vi "subpixel_maximum.vi"(1 "Padding":i32=3, 2 "Marginal":dbl[](graph)) -> (0 "Maximum":dbl format="%.2f")   [LabVIEW 2010]
panel:
  out "subpixel part":dbl(graph)
  out "max":dbl(graph)
  out "extracted region":dbl[](graph)
  out "alpha":dbl
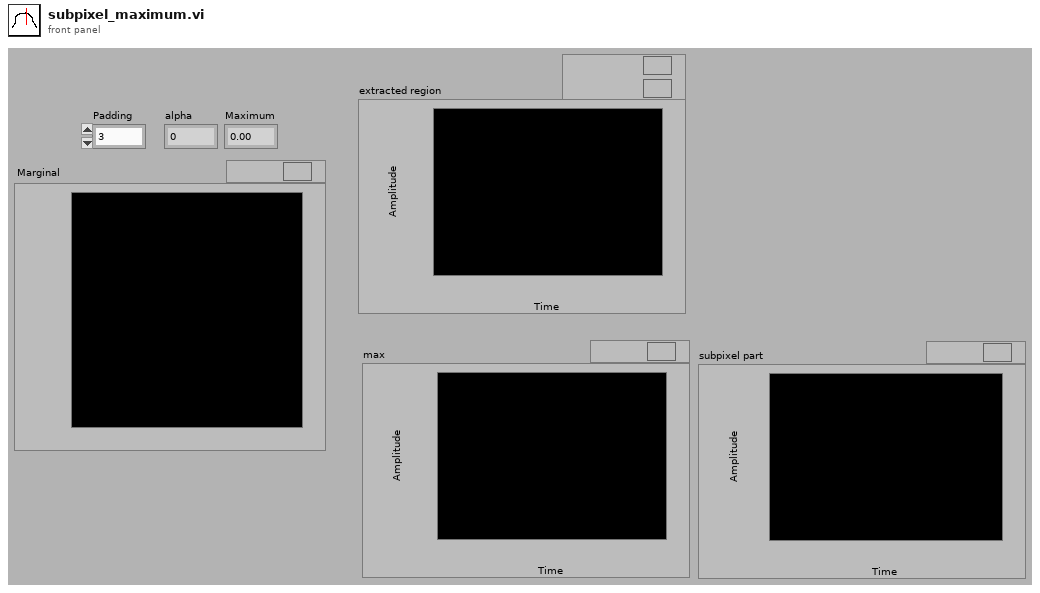
[diagram p1: front panel]
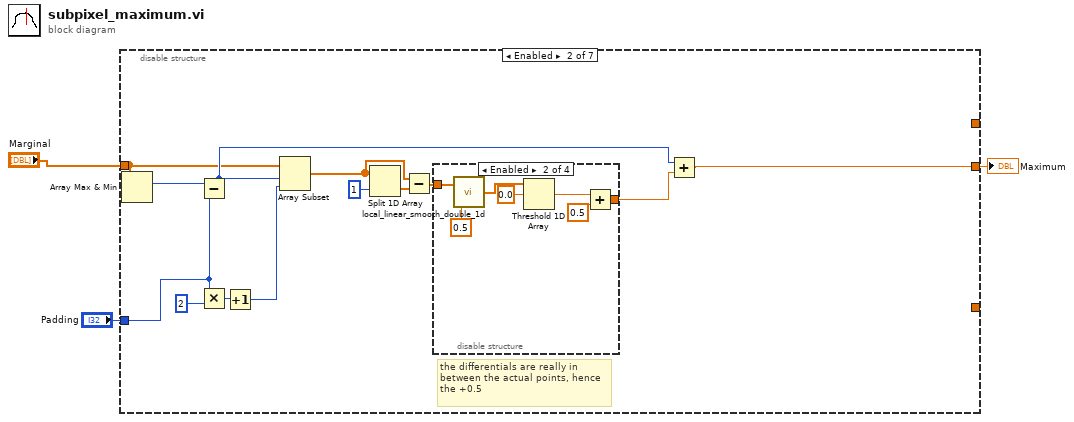
[diagram p0: block diagram]
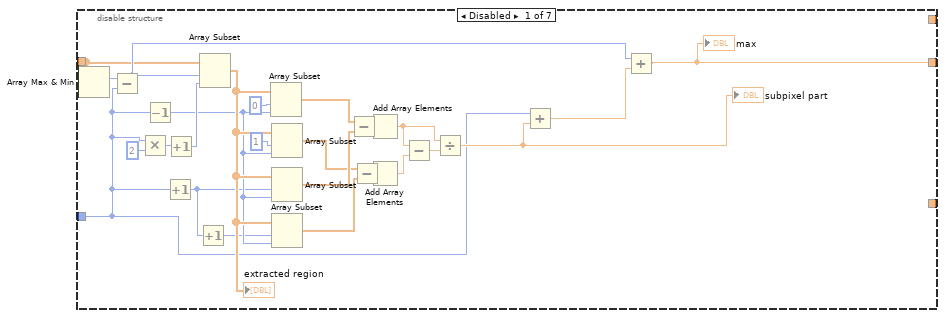
[diagram p2: hidden frame]
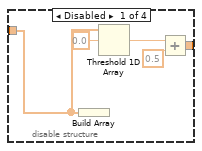
[diagram p3: hidden frame]
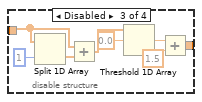
[diagram p4: hidden frame]
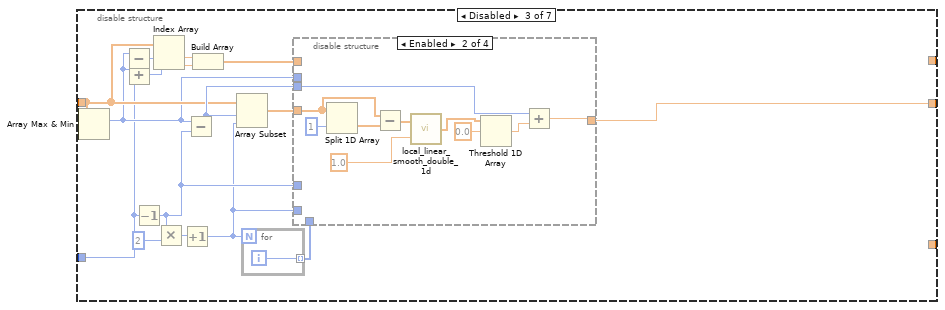
[diagram p6: hidden frame]
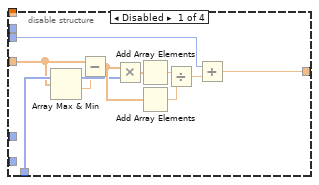
[diagram p7: hidden frame]
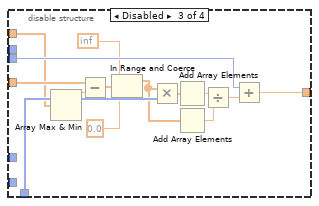
[diagram p8: hidden frame]
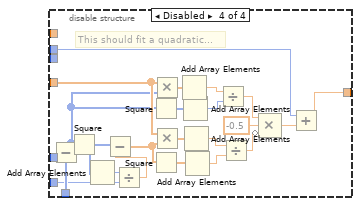
[diagram p9: hidden frame]
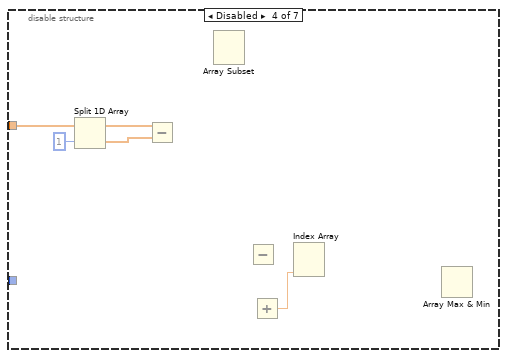
[diagram p10: hidden frame]
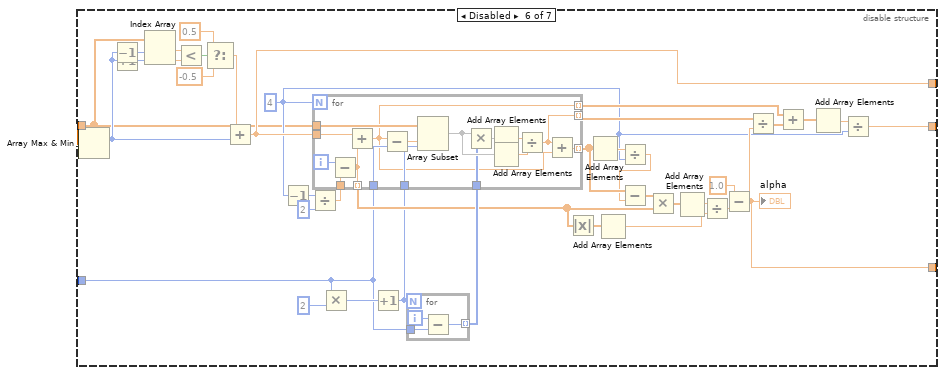
[diagram p12: hidden frame]
diagram:
  n1 = disable-structure shown="Enabled" {
    disable-tunnel: [w22 w29 w78 _ _ w142 _] -> w2
    disable-tunnel: "Marginal" -> [w25 w38 w72 w138 _ w141 _]
    disable-tunnel: "Padding" -> [w4 w33 w65 _ _ w152 _]
    disable-tunnel: [_ _ _ _ _ w155 _] -> _
    disable-tunnel: [_ _ _ _ _ w148 _] -> _
    frame Disabled {
      n2 = Array Max & Min(array=w25) -> (max index (indices)=w24:i32)  [unwired: 3 out]
      n3 = Subtract(x=w24, y=w4) -> (x-y=w28:i32)
      n4 = Multiply(x=w4, y=2) -> (x*y=w26:i32)
      n5 = Decrement(x=w4) -> (x-1=w18:i32)
      n6 = Increment(x=w4) -> (x+1=w16:i32)
      n7 = Increment(x=w26) -> (x+1=w23:i32)
      n8 = Increment(x=w16) -> (x+1=w17:i32)
      n9 = Array Subset(array=w25, index=w28, length=w23) -> (w19:dbl[])
      "extracted region" <- w19
      n10 = Array Subset(array=w19, index=0, length=w18) -> (w15:dbl[])
      n11 = Array Subset(array=w19, index=1, length=w18) -> (w13:dbl[])
      n12 = Array Subset(array=w19, index=w16, length=w18) -> (w14:dbl[])
      n13 = Array Subset(array=w19, index=w17, length=w18) -> (w12:dbl[])
      n14 = Subtract(x=w15, y=w14) -> (x-y=w9:dbl[])
      n15 = Subtract(x=w13, y=w12) -> (x-y=w11:dbl[])
      n16 = Add Array Elements(numeric array=w9) -> (sum=w8:dbl)
      n17 = Add Array Elements(numeric array=w11) -> (sum=w7:dbl)
      n18 = Subtract(x=w8, y=w7) -> (x-y=w10:dbl)
      n19 = Divide(x=w8, y=w10) -> (x/y=w6:dbl)
      "subpixel part" <- w6
      n20 = Add(x=w4, y=w6) -> (x+y=w5:dbl)
      n21 = Add(x=w28, y=w5) -> (x+y=w22:dbl)
      "max" <- w22
    }
    frame Enabled {
      # "the differentials are really in between the actual points, hence the +0.5"
      n22 = Array Max & Min(array=w38) -> (max index (indices)=w37:i32)  [unwired: 3 out]
      n23 = Subtract(x=w37, y=w33) -> (x-y=w41:i32)
      n24 = Multiply(x=w33, y=2) -> (x*y=w39:i32)
      n25 = Increment(x=w39) -> (x+1=w36:i32)
      n26 = Array Subset(array=w38, index=w41, length=w36) -> (w30:dbl[])
      n27 = Split 1D Array(array=w30, index=1) -> (second subarray=w34:dbl[])  [unwired: 1 out]
      n28 = Subtract(x=w30, y=w34) -> (x-y=w31:dbl[])
      n29 = disable-structure shown="Enabled" {
        disable-tunnel: w31 -> [w44 w51 w56 _]
        disable-tunnel: [w42 w49 w59 _] -> w32
        frame Disabled {
          n30 = Build Array(w44) -> (w46:dbl[][])
          n31 = Threshold 1D Array(2:0.0 ("threshold y"), 3:w44) -> (0:w43:dbl)  [unwired: 1 out]
          n32 = Add(x=w43, y=0.5) -> (x+y=w42:dbl)
        }
        frame Enabled {
          n33 = call "local_linear_smooth_double_1d.vi"("Smoothing Parameter (Gaussian S.D. in pixels)"=0.5, "Input Array"=w51) -> ("Smoothed Array"=w48:dbl[])
          n34 = Threshold 1D Array(2:0.0 ("threshold y"), 3:w48) -> (0:w50:dbl)  [unwired: 1 out]
          n35 = Add(x=w50, y=0.5) -> (x+y=w49:dbl)
        }
        frame Disabled {
          n36 = Split 1D Array(array=w56, index=1) -> (second subarray=w58:dbl[])  [unwired: 1 out]
          n37 = Add(x=w56, y=w58) -> (x+y=w55:dbl[])
          n38 = Threshold 1D Array(2:0.0 ("threshold y"), 3:w55) -> (0:w60:dbl)  [unwired: 1 out]
          n39 = Add(x=w60, y=1.5) -> (x+y=w59:dbl)
        }
        frame Disabled {
        }
      }
      n40 = Add(x=w41, y=w32) -> (x+y=w29:dbl)
    }
    frame Disabled {
      n41 = Array Max & Min(array=w72) -> (max index (indices)=w71:i32)  [unwired: 3 out]
      n42 = Subtract(x=w71, y=w65) -> (x-y=w70:i32)
      n43 = Add(x=w71, y=w65) -> (x+y=w69:i32)
      n44 = Decrement(x=w65) -> (x-1=w64:i32)
      n45 = Index Array(array=w72, index #1=w70, index #2=w69) -> (element #1=w67:dbl, element #2=w68:dbl)
      n46 = Multiply(x=w64, y=2) -> (x*y=w73:i32)
      n47 = Increment(x=w73) -> (x+1=w63:i32)
      n48 = Subtract(x=w71, y=w64) -> (x-y=w77:i32)
      n49 = Build Array(w67, w68) -> (w66:dbl[])
      n50 = Array Subset(array=w72, index=w77, length=w63) -> (w75:dbl[])
      n51 = for {
        N: w63 -> [_]
        tunnel: [w136] -> w76 mode=indexing
        i -> [w136]
      }
      n52 = disable-structure shown="Enabled" {
        disable-tunnel: [w88 w98 w112 w123] -> w78
        disable-tunnel: w77 -> [w87 w97 w111 _]
        disable-tunnel: w76 -> [w81 _ w106 w121]
        disable-tunnel: w75 -> [w80 w94 w105 w135]
        disable-tunnel: w71 -> [_ _ _ w124]
        disable-tunnel: w64 -> [_ _ _ w120]
        disable-tunnel: w66 -> [_ _ w104 _]
        disable-tunnel: w63 -> [_ _ _ w116]
        frame Disabled {
          n53 = Array Max & Min(array=w80) -> (min value=w79:dbl)  [unwired: 3 out]
          n54 = Subtract(x=w80, y=w79) -> (x-y=w82:dbl[])
          n55 = Multiply(x=w82, y=w81) -> (x*y=w84:dbl[])
          n56 = Add Array Elements(numeric array=w84) -> (sum=w85:dbl)
          n57 = Add Array Elements(numeric array=w82) -> (sum=w83:dbl)
          n58 = Divide(x=w85, y=w83) -> (x/y=w86:dbl)
          n59 = Add(x=w87, y=w86) -> (x+y=w88:dbl)
        }
        frame Enabled {
          n60 = Split 1D Array(array=w94, index=1) -> (second subarray=w95:dbl[])  [unwired: 1 out]
          n61 = Subtract(x=w94, y=w95) -> (x-y=w91:dbl[])
          n62 = call "local_linear_smooth_double_1d.vi"("Smoothing Parameter (Gaussian S.D. in pixels)"=1.0, "Input Array"=w91) -> ("Smoothed Array"=w90:dbl[])
          n63 = Threshold 1D Array(2:0.0 ("threshold y"), 3:w90) -> (0:w92:dbl)  [unwired: 1 out]
          n64 = Add(x=w97, y=w92) -> (x+y=w98:dbl)
        }
        frame Disabled {
          n65 = Array Max & Min(array=w104) -> (max value=w103:dbl)  [unwired: 3 out]
          n66 = Subtract(x=w105, y=w103) -> (x-y=w102:dbl[])
          n67 = In Range and Coerce(upper limit=inf, x=w102, lower limit=sgl 0.0) -> (coerced(x)=w101:dbl[])  [unwired: 1 out]
          n68 = Multiply(x=w101, y=w106) -> (x*y=w108:dbl[])
          n69 = Add Array Elements(numeric array=w108) -> (sum=w109:dbl)
          n70 = Add Array Elements(numeric array=w101) -> (sum=w107:dbl)
          n71 = Divide(x=w109, y=w107) -> (x/y=w110:dbl)
          n72 = Add(x=w111, y=w110) -> (x+y=w112:dbl)
        }
        frame Disabled {
          # "This should fit a quadratic..."
          n73 = Subtract(x=w121, y=w120) -> (x-y=w122:i32[])
          n74 = Square(x=w122) -> (x^2=w115:i32[])
          n75 = Add Array Elements(numeric array=w115) -> (sum=w117:i32)
          n76 = Divide(x=w117, y=w116) -> (x/y=w118:dbl)
          n77 = Subtract(x=w115, y=w118) -> (x-y=w114:dbl[])
          n78 = Square(x=w122) -> (x^2=w133:i32[])
          n79 = Square(x=w114) -> (x^2=w131:dbl[])
          n80 = Multiply(x=w135, y=w122) -> (x*y=w134:dbl[])
          n81 = Multiply(x=w135, y=w114) -> (x*y=w132:dbl[])
          n82 = Add Array Elements(numeric array=w134) -> (sum=w128:dbl)
          n83 = Add Array Elements(numeric array=w133) -> (sum=w129:i32)
          n84 = Add Array Elements(numeric array=w132) -> (sum=w113:dbl)
          n85 = Add Array Elements(numeric array=w131) -> (sum=w130:dbl)
          n86 = Divide(x=w128, y=w129) -> (x/y=w127:dbl)
          n87 = Divide(x=w113, y=w130) -> (x/y=w126:dbl)
          n88 = Compound Arithmetic op=MULTIPLY(w127, sgl -0.5 ("value"), invert w126) -> (w119:dbl)
          n89 = Add(x=w124, y=w119) -> (x+y=w123:dbl)
        }
      }
    }
    frame Disabled {
      n90 = Split 1D Array(array=w138, index=1) -> (second subarray=w139:dbl[])  [unwired: 1 out]
      n91 = Subtract(x=w138, y=w139) -> ()  [unwired: 1 out]
      n92 = Array Subset() -> ()  [unwired: 3 in, 1 out]
      n93 = Subtract() -> ()  [unwired: 2 in, 1 out]
      n94 = Add() -> (x+y=w137:dbl)  [unwired: 2 in]
      n95 = Index Array(index #2=w137) -> ()  [unwired: 2 in, 2 out]
      n96 = Array Max & Min() -> ()  [unwired: 1 in, 4 out]
    }
    frame Disabled {
    }
    frame Disabled {
      w143 = 4
      n97 = Array Max & Min(array=w141) -> (max index (indices)=w173:i32)  [unwired: 3 out]
      n98 = Decrement(x=w173) -> (x-1=w177:i32)
      n99 = Increment(x=w173) -> (x+1=w176:i32)
      n100 = Index Array(array=w141, index #1=w177, index #2=w176) -> (element #1=w175:dbl, element #2=w174:dbl)
      n101 = Less?(x=w175, y=w174) -> (x < y?=w159:bool)
      n102 = Select(t=0.5 ("x"), s=w159, f=-0.5 ("x")) -> (s? t:f=w156:dbl)
      n103 = Add(x=w156, y=w173) -> (x+y=w155:dbl)
      n104 = Decrement(x=w143) -> (x-1=w169:i32)
      n105 = Divide(x=w169, y=2) -> (x/y=w154:dbl)
      n106 = Multiply(x=w152, y=2) -> (x*y=w172:i32)
      n107 = Increment(x=w172) -> (x+1=w151:i32)
      n108 = for {
        N: w151 -> [_]
        tunnel: [w195] -> w171 mode=indexing
        tunnel: w152 -> [w196]
        i -> [w197]
        n109 = Subtract(x=w197, y=w196) -> (x-y=w195:i32)
      }
      n110 = for {
        N: w143 -> [_]
        tunnel: w141 -> [w190]
        tunnel: w155 -> [w189]
        tunnel: w151 -> [w188]
        tunnel: w171 -> [w187]
        tunnel: [w186] -> w165 mode=indexing
        tunnel: w154 -> [w184]
        tunnel: w152 -> [w182]
        tunnel: [w181] -> w153 mode=indexing
        tunnel: [w180] -> w149 mode=indexing
        tunnel: [w179] -> w146 mode=indexing
        i -> [w185]
        n111 = Subtract(x=w185, y=w184) -> (x-y=w181:dbl)
        n112 = Add(x=w189, y=w181) -> (x+y=w179:dbl)
        n113 = Subtract(x=w179, y=w182) -> (x-y=w183:dbl)
        n114 = Array Subset(array=w190, index=w183, length=w188) -> (w194:dbl[])
        n115 = Multiply(x=w194, y=w187) -> (x*y=w192:dbl[])
        n116 = Add Array Elements(numeric array=w192) -> (sum=w191:dbl)
        n117 = Add Array Elements(numeric array=w194) -> (sum=w193:dbl)
        n118 = Divide(x=w191, y=w193) -> (x/y=w180:dbl)
        n119 = Add(x=w180, y=w179) -> (x+y=w186:dbl)
      }
      n120 = Absolute Value(x=w153) -> (abs(x)=w161:dbl[])
      n121 = Add Array Elements(numeric array=w165) -> (sum=w170:dbl)
      n122 = Add Array Elements(numeric array=w161) -> (sum=w160:dbl)
      n123 = Divide(x=w170, y=w143) -> (x/y=w150:dbl)
      n124 = Subtract(x=w165, y=w150) -> (x-y=w166:dbl[])
      n125 = Multiply(x=w166, y=w153) -> (x*y=w167:dbl[])
      n126 = Add Array Elements(numeric array=w167) -> (sum=w164:dbl)
      n127 = Divide(x=w164, y=w160) -> (x/y=w163:dbl)
      n128 = Subtract(x=1.0, y=w163) -> (x-y=w148:dbl)
      "alpha" <- w148
      n129 = Divide(x=w149, y=w148) -> (x/y=w147:dbl[])
      n130 = Add(x=w146, y=w147) -> (x+y=w144:dbl[])
      n131 = Add Array Elements(numeric array=w144) -> (sum=w145:dbl)
      n132 = Divide(x=w145, y=w143) -> (x/y=w142:dbl)
    }
    frame Disabled {
    }
  }
  "Maximum" <- w2
